vi "Attempt to resolve locally.vi"(8 "error in (no error)":errorcluster, 11 "address":refnum<class "Generic Network Address.lvclass">) -> (0 "error out":errorcluster, 3 "addresses out":refnum<class "Generic Network Address.lvclass">[](array[class]))   [LabVIEW 2020, in "NI_WFCN.lvlib" / "Generic Network Address.lvclass"]
doc: "Use local facilities to resolve this address into the address which should be resolved next. For IP addresses, this typically does nothing. If a hostname is in /etc/hosts, this will look up its IP and return it. For DNS hostnames, this will return a DNS nameserver IP."
uses:
  <vilib>/net/WFCN/Addressing/Generic Network Address/Generic Network Address.lvclass
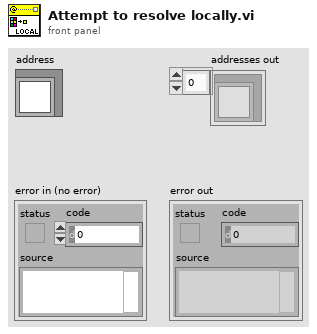
[diagram p1: front panel]
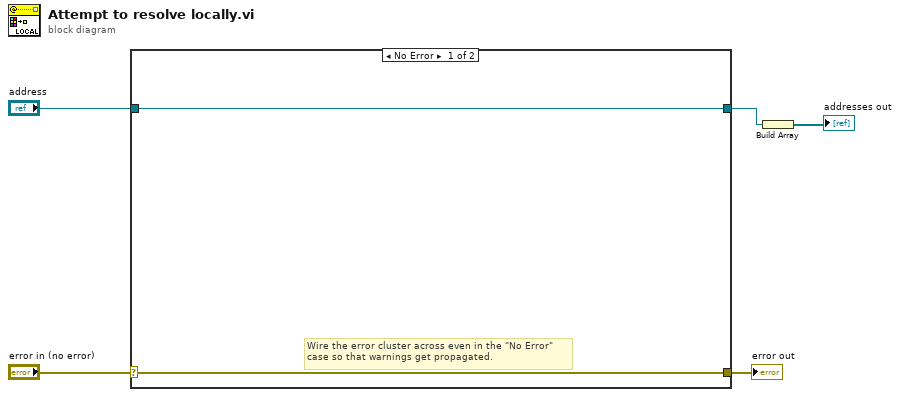
[diagram p0: block diagram]
diagram:
  n1 = case shown="No Error" "error in (no error)" {
    selector: "error in (no error)" -> [w6 w9]
    tunnel: [w6 w9] -> w4
    tunnel: [w7 w8] -> w2
    tunnel: "address" -> [w7 w8]
    frame No Error {
      # "Wire the error cluster across even in the \"No Error\"\ncase so that warnings get propagated."
    }
    frame Error {
    }
  }
  "error out" <- w4
  n2 = Build Array(w2) -> (→"addresses out":refnum<class "Generic Network Address.lvclass">[])
